vi "Columns.vi"() -> (2 "Columns":T1)   [LabVIEW 2022 SP3, in "Test.lvlib" / "User.lvclass"]
uses:
  User.lvclass
  Columns.ctl
  <vilib>/IlluminatedG/IG Conditum/Conditum/Columns/String/String.lvclass
  <vilib>/IlluminatedG/IG Conditum/Conditum/Columns/Timestamp/Timestamp.lvclass
  <vilib>/IlluminatedG/IG Conditum/Conditum/Columns/Boolean/Boolean.lvclass
  <vilib>/IlluminatedG/IG Conditum/Conditum/Columns/Integer/Integer.lvclass
  <vilib>/IlluminatedG/IG Conditum/Conditum/Columns/String/String Definition.ctl
  <vilib>/IlluminatedG/IG Conditum/Conditum/Columns/Type/Definition.ctl
  <vilib>/IlluminatedG/IG Conditum/Conditum/Attributes.ctl
  <vilib>/IlluminatedG/IG Conditum/Conditum/Columns/String/Definition.ctl
  <vilib>/IlluminatedG/IG Conditum/Conditum/Columns/Timestamp/DateTime Definition.ctl
  <vilib>/IlluminatedG/IG Conditum/Conditum/Columns/Timestamp/Definition.ctl
  <vilib>/IlluminatedG/IG Conditum/Conditum/Columns/Boolean/Boolean Definition.ctl
  <vilib>/IlluminatedG/IG Conditum/Conditum/Columns/Boolean/Definition.ctl
  <vilib>/IlluminatedG/IG Conditum/Conditum/Columns/Integer/Integer Definition.ctl
  <vilib>/IlluminatedG/IG Conditum/Conditum/Columns/Integer/Definition.ctl
  <vilib>/IlluminatedG/IG Conditum/Conditum/Conditum.lvlib
  <vilib>/IlluminatedG/IG Conditum/Conditum/Columns/Type/Type.lvclass
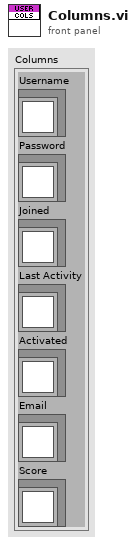
[diagram p1: front panel]
types:
  T1 = typedef "Test.lvlib/User.lvclass/Columns.ctl" = cluster{"Username":refnum<class "String.lvclass">, "Password":refnum<class "String.lvclass">, "Joined":refnum<class "Timestamp.lvclass">, "Last Activity":refnum<class "Timestamp.lvclass">, "Activated":refnum<class "Boolean.lvclass">, "Email":refnum<class "String.lvclass">, "Score":refnum<class "Integer.lvclass">}
  T2 = typedef "Conditum.lvlib/Columns.lvlib/Integer.lvclass/Integer Definition.ctl" = cluster{"Type":T3, "Attributes":T4, "Integer":T5}
  T3 = typedef "Conditum.lvlib/Columns.lvlib/Type.lvclass/Definition.ctl" = cluster{"Name":string, "Nullable":bool, "Default NULL":bool}
  T4 = typedef "Conditum.lvlib/Attributes.ctl" = cluster{"Primary Key":bool, "Unique":bool, "Foreign Key":bool, "Auto Increment":bool}
  T5 = typedef "Conditum.lvlib/Columns.lvlib/Integer.lvclass/Definition.ctl" = cluster{"Default":i64}
  T6 = typedef "Conditum.lvlib/Columns.lvlib/String.lvclass/String Definition.ctl" = cluster{"Type":T3, "Attributes":T4, "String":T7}
  T7 = typedef "Conditum.lvlib/Columns.lvlib/String.lvclass/Definition.ctl" = cluster{"Default":string, "Length":i32}
  T8 = typedef "Conditum.lvlib/Columns.lvlib/Boolean.lvclass/Boolean Definition.ctl" = cluster{"Type":T3, "Attributes":T4, "Boolean":T9}
  T9 = typedef "Conditum.lvlib/Columns.lvlib/Boolean.lvclass/Definition.ctl" = cluster{"Default":bool}
  T10 = typedef "Conditum.lvlib/Columns.lvlib/Timestamp.lvclass/DateTime Definition.ctl" = cluster{"Type":T3, "Attributes":T4, "DateTime":T11}
  T11 = typedef "Conditum.lvlib/Columns.lvlib/Timestamp.lvclass/Definition.ctl" = cluster{"Default":timestamp}
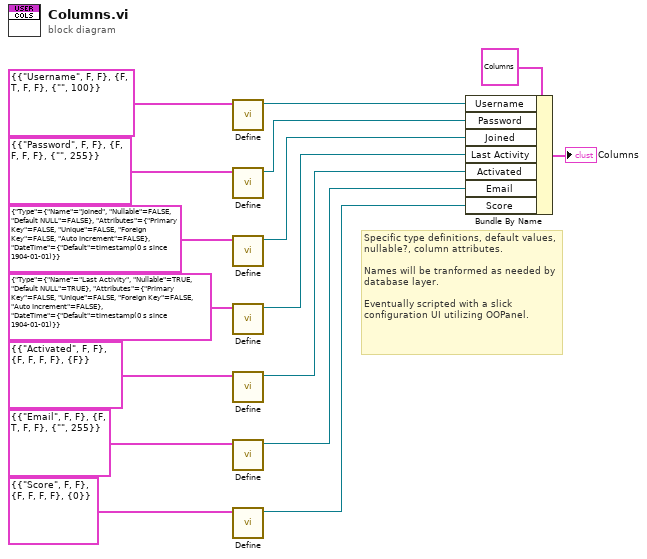
[diagram p0: block diagram]
diagram:
  # "Specific type definitions, default values, nullable?, column attributes.\n\nNames will be tranformed as needed by database layer.\n\nEventually scripted with a slick configuration UI utilizing OOPanel."
  n1 = call <vilib>:"Define.vi"("Definition"=T6 {"Type"={"Name"="Username", "Nullable"=FALSE, "Default NULL"=FALSE}, "Attributes"={"Primary Key"=FALSE, "Unique"=TRUE, "Foreign Key"=FALSE, "Auto Increment"=FALSE}, "String"={"Default"="", "Length"=100}}) -> ("String out"=w13:refnum<class "String.lvclass">)  [unwired: 10 in]
  n2 = call <vilib>:"Define.vi"("Definition"=T6 {"Type"={"Name"="Password", "Nullable"=FALSE, "Default NULL"=FALSE}, "Attributes"={"Primary Key"=FALSE, "Unique"=FALSE, "Foreign Key"=FALSE, "Auto Increment"=FALSE}, "String"={"Default"="", "Length"=255}}) -> ("String out"=w12:refnum<class "String.lvclass">)  [unwired: 10 in]
  n3 = call <vilib>:"Define.vi"("Definition"=T10 {"Type"={"Name"="Joined", "Nullable"=FALSE, "Default NULL"=FALSE}, "Attributes"={"Primary Key"=FALSE, "Unique"=FALSE, "Foreign Key"=FALSE, "Auto Increment"=FALSE}, "DateTime"={"Default"=timestamp(0 s since 1904-01-01)}}) -> ("DateTime out"=w9:refnum<class "Timestamp.lvclass">)  [unwired: 10 in]
  n4 = call <vilib>:"Define.vi"("Definition"=T10 {"Type"={"Name"="Last Activity", "Nullable"=TRUE, "Default NULL"=TRUE}, "Attributes"={"Primary Key"=FALSE, "Unique"=FALSE, "Foreign Key"=FALSE, "Auto Increment"=FALSE}, "DateTime"={"Default"=timestamp(0 s since 1904-01-01)}}) -> ("DateTime out"=w7:refnum<class "Timestamp.lvclass">)  [unwired: 10 in]
  n5 = call <vilib>:"Define.vi"("Init Data"=T8 {"Type"={"Name"="Activated", "Nullable"=FALSE, "Default NULL"=FALSE}, "Attributes"={"Primary Key"=FALSE, "Unique"=FALSE, "Foreign Key"=FALSE, "Auto Increment"=FALSE}, "Boolean"={"Default"=FALSE}}) -> ("Boolean out"=w5:refnum<class "Boolean.lvclass">)  [unwired: 10 in]
  n6 = call <vilib>:"Define.vi"("Definition"=T6 {"Type"={"Name"="Email", "Nullable"=FALSE, "Default NULL"=FALSE}, "Attributes"={"Primary Key"=FALSE, "Unique"=TRUE, "Foreign Key"=FALSE, "Auto Increment"=FALSE}, "String"={"Default"="", "Length"=255}}) -> ("String out"=w3:refnum<class "String.lvclass">)  [unwired: 10 in]
  n7 = call <vilib>:"Define.vi"("Integer Definition"=T2 {"Type"={"Name"="Score", "Nullable"=FALSE, "Default NULL"=FALSE}, "Attributes"={"Primary Key"=FALSE, "Unique"=FALSE, "Foreign Key"=FALSE, "Auto Increment"=FALSE}, "Integer"={"Default"=0}}) -> ("Integer out"=w1:refnum<class "Integer.lvclass">)  [unwired: 10 in]
  n8 = Bundle By Name(cluster=T1 {"Username"=refnum, "Password"=refnum, "Joined"=refnum, "Last Activity"=refnum, "Activated"=refnum, "Email"=refnum, "Score"=refnum} ("Columns"), "Username"=w13, "Password"=w12, "Joined"=w9, "Last Activity"=w7, "Activated"=w5, "Email"=w3, "Score"=w1) -> (→"Columns":T1)
